vi "sortChannelOutputState.vi"(8 "error in (no error)":errorcluster, 9 "calibratedValues":dbl[](array[numeric]), 10 "channel_addresses":string[](array[string]), 11 "DigitalOutput in":refnum<class "DigitalOutput.lvclass">) -> (0 "error out":errorcluster, 1 "calibratedValues out":dbl[](array[numeric]), 2 "channel_addresses out":string[](array[string]), 3 "DigitalOutput out":refnum<class "DigitalOutput.lvclass">)   [LabVIEW 2009, in "Hardware.lvlib" / "Channels.lvlib" / "DigitalOutput.lvclass"]
uses:
  DigitalOutput.lvclass
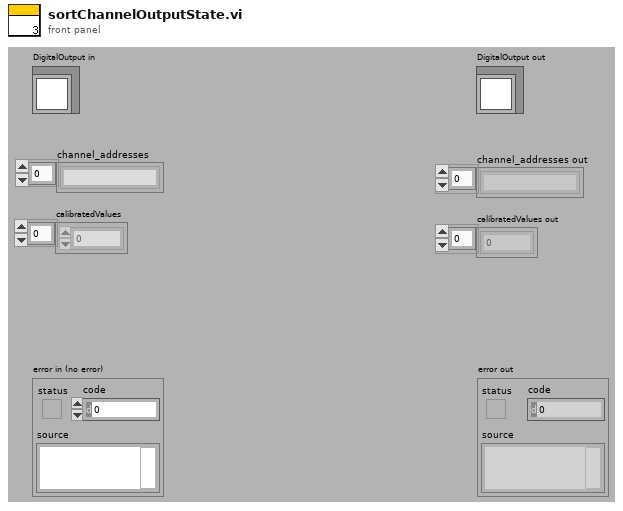
[diagram p1: front panel]
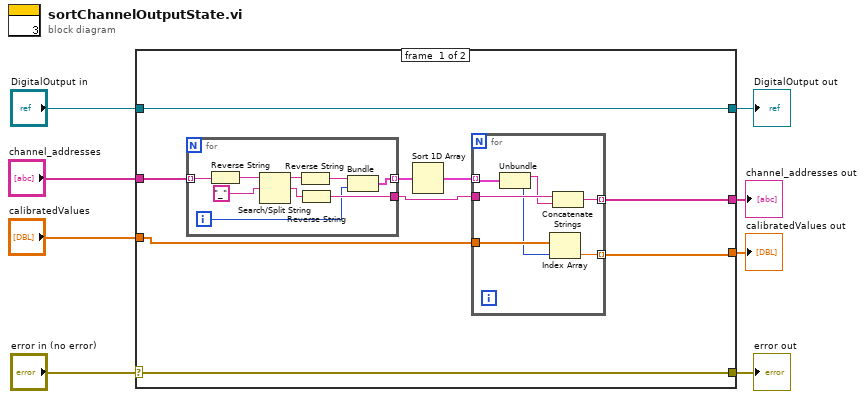
[diagram p0: block diagram]
diagram:
  n1 = case shown="No Error" "error in (no error)" {
    selector: "error in (no error)" -> [w16 w35]
    tunnel: [w16 w35] -> w7
    tunnel: [w17 w34] -> w5
    tunnel: "DigitalOutput in" -> [w17 w34]
    tunnel: "channel_addresses" -> [w15 _]
    tunnel: "calibratedValues" -> [w12 _]
    tunnel: [w10 _] -> w2
    tunnel: [w9 _] -> w1
    frame #0 {
      n2 = for {
        tunnel: w15 -> [w33] mode=indexing
        tunnel: [w28] -> w11
        tunnel: [w25] -> w14 mode=indexing
        i -> [w26]
        n3 = Reverse String(1:w33) -> (0:w32:string)
        n4 = Search/Split String(string=w32, search string/char (-)="_") -> (substring before match=w30:string, match + rest of string=w29:string)  [unwired: 1 in, 1 out]
        n5 = Reverse String(1:w30) -> (0:w27:string)
        n6 = Reverse String(1:w29) -> (0:w28:string)
        n7 = Bundle(w27, w26) -> (w25:cluster{string, i32})  [unwired: 1 in]
      }
      n8 = Sort 1D Array(array=w14) -> (sorted array=w13:cluster{string, i32}[])
      n9 = for {
        tunnel: w13 -> [w24] mode=indexing
        tunnel: w12 -> [w20]
        tunnel: w11 -> [w23]
        tunnel: [w21] -> w10 mode=indexing
        tunnel: [w18] -> w9 mode=indexing
        n10 = Unbundle(w24) -> (w22:string, w19:i32)
        n11 = Index Array(array=w20, index=w19) -> (element=w18:dbl)
        n12 = Concatenate Strings(w23, w22) -> (w21:string)
      }
    }
    frame #1 {
    }
  }
  "error out" <- w7
  "DigitalOutput out" <- w5
  "channel_addresses out" <- w2
  "calibratedValues out" <- w1
